vi "Ball_Collector.vi"   [LabVIEW 2011]
uses:
  StateMachineType.ctl
  <vilib>/Rock Robotics/WPI/Relay/WPI_RelayValue.ctl
  Robot Global Data.vi
types:
  T1 = typedef "StateMachineType.ctl" = enum16{"Init", "Idle", "Start", "Do", "Stop"}
  T2 = typedef "WPI_RelayValue.ctl" = enum16{"Off", "On", "Forward", "Reverse"}
  T3 = typedef "WPI_RelayDevRef.ctl" = cluster{"DevStatus":errorcluster, "Relay Channel":T4, "Digital Module":T5, "Relay Direction":T6}
  T4 = typedef "FPGA_DIORelayChannel.ctl" = enum8{"Relay 1", "Relay 2", "Relay 3", "Relay 4", "Relay 5", "Relay 6", "Relay 7", "Relay 8", "Invalid"}
  T5 = typedef "FPGA_TypedefDigitalModule.ctl" = enum16{"Digital Module 1", "Digital Module 2"}
  T6 = typedef "WPI_RelayDirection.ctl" = enum16{"Both directions", "Forward only", "Reverse only"}
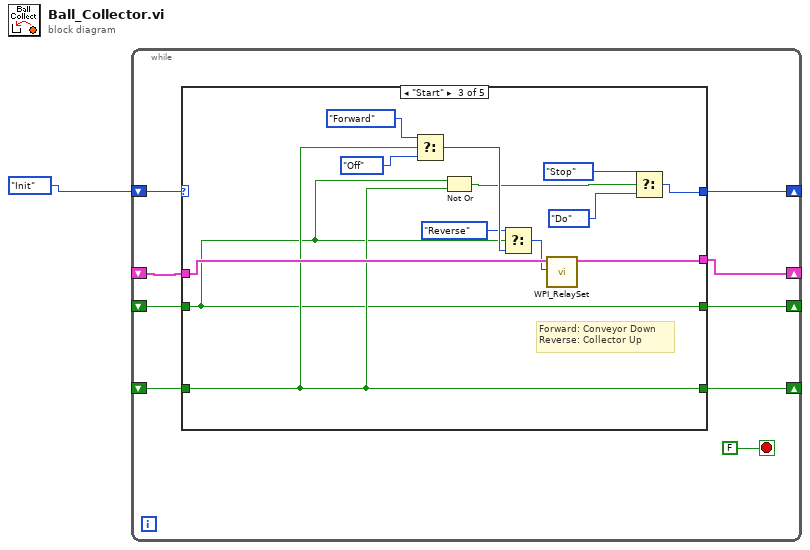
[diagram p0: block diagram]
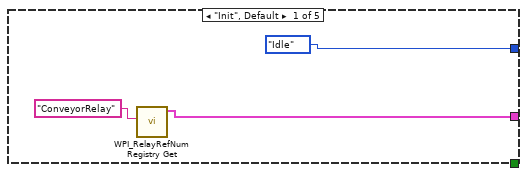
[diagram p2: hidden frame]
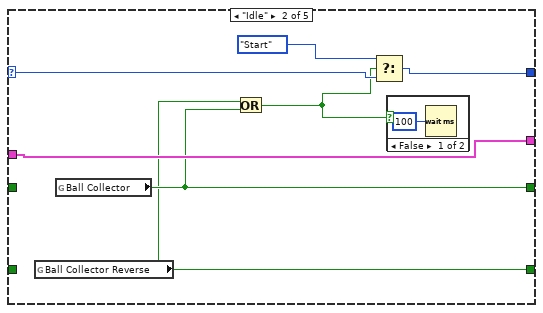
[diagram p3: hidden frame]
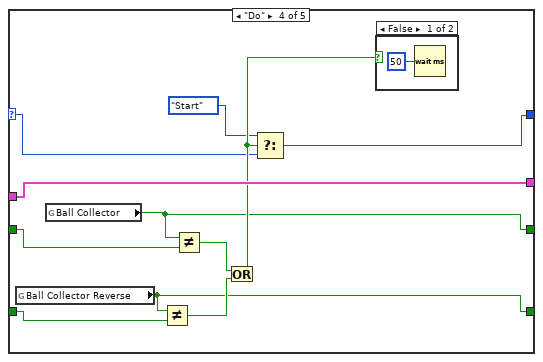
[diagram p5: hidden frame]
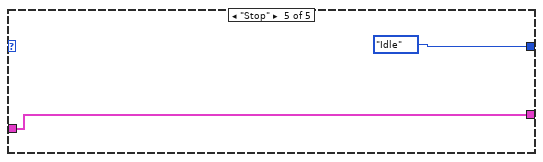
[diagram p7: hidden frame]
diagram:
  n1 = while {
    shift-right: [w6] -> _
    shift-left: _ -> [w9]
    shift-right: [w7] -> _
    shift-left: StateMachineType."Init" -> [w8]
    shift-right: [w4] -> _
    shift-left: _ -> [w2]
    shift-right: [w5] -> _
    shift-left: _ -> [w3]
    stop <- FALSE stop-if-true
    n2 = case shown="\"Start\"" w8 {
      selector: w8 -> [_ w20 _ w35 _]
      tunnel: w9 -> [_ w17 w34 w45 w47]
      tunnel: [StateMachineType."Idle" ("Enum") w18 w26 w39 StateMachineType."Idle" ("Enum")] -> w7
      tunnel: [w11 w17 w33 w45 w47] -> w6
      tunnel: [_ w15 w23 w38 _] -> w5
      tunnel: [_ w14 w24 w37 _] -> w4
      tunnel: w3 -> [_ _ w23 w44 _]
      tunnel: w2 -> [_ _ w24 w43 _]
      frame "Init", Default {
        n3 = call <vilib>:"WPI_RelayRefNum Registry Get.vi"("refnum name"="ConveyorRelay") -> ("RelayDevRef"=w11:T3)  [unwired: 9 in, 1 out]
      }
      frame "Idle" {
        n4 = global read "Robot Global Data.vi" "Ball Collector Reverse"() -> (w14:bool)
        n5 = global read "Robot Global Data.vi" "Ball Collector"() -> (w15:bool)
        n6 = Or(x=w14, y=w15) -> (x .or. y?=w16:bool)
        n7 = Select(t=StateMachineType."Start" ("Enum"), s=w16, f=w20) -> (s? t:f=w18:T1)
        n8 = case shown="False" w16 {
          frame False {
            n9 = Wait (ms)(milliseconds to wait=u32 100) -> ()  [unwired: 1 out]
          }
          frame True {
          }
        }
      }
      frame "Start" {
        # "Forward: Conveyor Down\nReverse: Collector Up"
        n10 = Select(t=WPI_RelayValue."Forward" ("RelayValue"), s=w24, f=WPI_RelayValue."Off" ("RelayValue")) -> (s? t:f=w30:T2)
        n11 = Not Or(1:w24, 2:w23) -> (0:w25:bool)
        n12 = Select(t=WPI_RelayValue."Reverse", s=w23, f=w30) -> (s? t:f=w29:T2)
        n13 = call <vilib>:"WPI_RelaySet.vi"("RelayValue"=w29, "RelayDevRef"=w34) -> ("RelayDevRef"=w33:T3)  [unwired: 8 in, 1 out]
        n14 = Select(t=StateMachineType."Stop" ("Enum"), s=w25, f=StateMachineType."Do" ("Enum")) -> (s? t:f=w26:T1)
      }
      frame "Do" {
        n15 = global read "Robot Global Data.vi" "Ball Collector Reverse"() -> (w37:bool)
        n16 = global read "Robot Global Data.vi" "Ball Collector"() -> (w38:bool)
        n17 = Not Equal?(x=w37, y=w43) -> (x != y?=w41:bool)
        n18 = Not Equal?(x=w38, y=w44) -> (x != y?=w42:bool)
        n19 = Or(x=w42, y=w41) -> (x .or. y?=w40:bool)
        n20 = Select(t=StateMachineType."Start" ("Enum"), s=w40, f=w35) -> (s? t:f=w39:T1)
        n21 = case shown="False" w40 {
          frame False {
            n22 = Wait (ms)(milliseconds to wait=u32 50) -> ()  [unwired: 1 out]
          }
          frame True {
          }
        }
      }
      frame "Stop" {
      }
    }
  }
